vi "Wave-Open File.vi"(8 "error in (no error)":errorcluster, 11 "Path":path) -> (0 "error out":errorcluster, 3 "refnum out":refnum<file>)   [LabVIEW 2020]
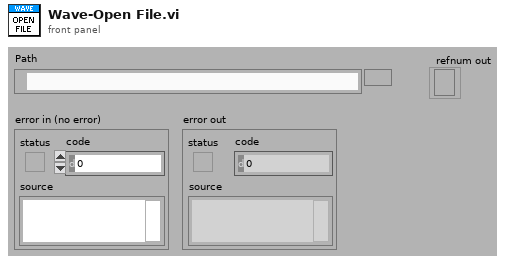
[diagram p1: front panel]
types:
  T1 = enum16{"open", "replace", "create", "open or create", "replace or create", "replace or create with confirmation"}
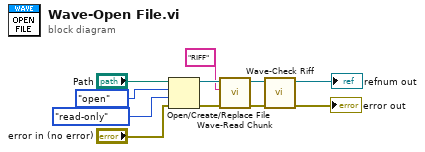
[diagram p0: block diagram]
diagram:
  n1 = Open/Create/Replace File(file path (use dialog)="Path", error in="error in (no error)", operation (0:open)=T1."open", access (0:read/write)=enum16{"read/write", "read-only", "write-only"}."read-only") -> (refnum out=w5:refnum<file>, error out=w6:errorcluster)  [unwired: 2 in, 1 out]
  n2 = call "Wave-Read Chunk.vi"("error in (no error)"=w6, "ID"="RIFF", "refnum"=w5) -> ("error out"=w4:errorcluster, "refnum out"=w3:refnum<file>)  [unwired: 5 in, 2 out]
  n3 = call "Wave-Check Riff.vi"("error in (no error)"=w4, "refnum"=w3) -> ("error out"=→"error out":errorcluster, "refnum out"=→"refnum out":refnum<file>)  [unwired: 7 in, 1 out]
